vi "Read Status.vi"(8 "error in (no error)":errorcluster, 11 "CV-Main in":refnum<class "CV-Main.lvclass">) -> (0 "error out":errorcluster, 2 "Status":T1, 3 "CV-Main out":refnum<class "CV-Main.lvclass">)   [LabVIEW 2013, in "CameraVision.lvlib" / "CV-Main.lvclass"]
uses:
  CV-Main.lvclass
  Application-states.ctl
  CV-Main.lvclass/CV-Main.ctl
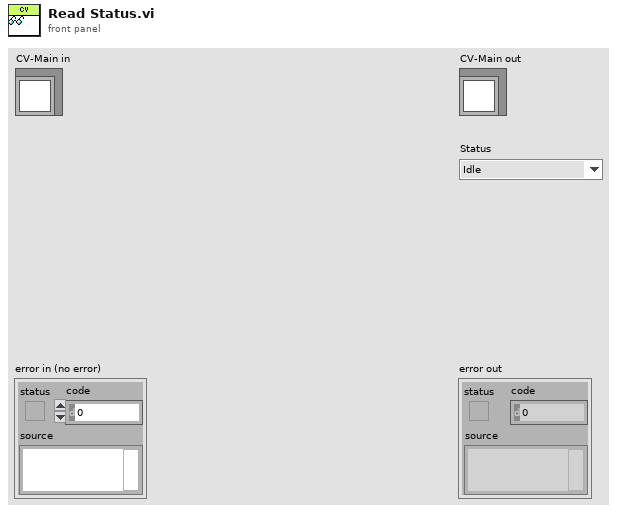
[diagram p1: front panel]
types:
  T1 = typedef "CameraVision.lvlib/CV-Main.lvclass/Application-states.ctl" = enum16{"Idle", "Initialized", "Configured", "Activated", "Started", "Stopped", "Reset", "Error", "Exited"}
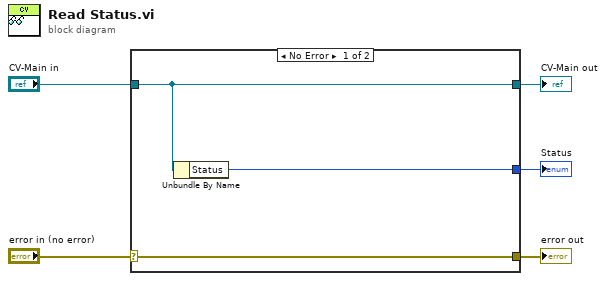
[diagram p0: block diagram]
diagram:
  n1 = case shown="No Error" "error in (no error)" {
    selector: "error in (no error)" -> [w8 w9]
    tunnel: [w8 w9] -> w4
    tunnel: [w7 w10] -> w2
    tunnel: "CV-Main in" -> [w7 w10]
    tunnel: [w6 _] -> w1
    frame No Error {
      n2 = Unbundle By Name(w7) -> ("Status"=w6:T1)
    }
    frame Error {
    }
  }
  "error out" <- w4
  "CV-Main out" <- w2
  "Status" <- w1
